vi "~Graph Sequence test.vi"(10 "PAARD Test Seq":T1[](array[typedef])=[{"StepType"=enum."Motion", "RF In/Out"=enum."Rx - RF Out", "Module/Raster"=0, "Polarization"=enum."Horizontal", "AO-64 Array"=[], "Position"=[]}, {"StepType"=enum."RasterTest", "RF In/Out"=enum."Tx - RF In", "Module/Raster"=0, "Polarization"=enum."Vertical", "AO-64 Array"=[], "Position"=[]}, {"StepType"=enum."Motion", "RF In/Out"=enum."Rx - RF Out", "Module/Raster"=1, "Polarization"=enum."Horizontal", "AO-64 Array"=[], "Position"=[]}, {"StepType"=enum."RasterTest", "RF In/Out"=enum."Tx - RF In", "Module/Raster"=0, "Polarization"=enum."Vertical", "AO-64 Array"=[], "Position"=[]}, {"StepType"=enum."Motion", "RF In/Out"=enum."Rx - RF Out", "Module/Raster"=2, "Polarization"=enum."Horizontal", "AO-64 Array"=[], "Position"=[]}, {"StepType"=enum."RasterTest", "RF In/Out"=enum."Tx - RF In", "Module/Raster"=0, "Polarization"=enum."Vertical", "AO-64 Array"=[], "Position"=[]}, {"StepType"=enum."Motion", "RF In/Out"=enum."Rx - RF Out", "Module/Raster"=3, "Polarization"=enum."Horizontal", "AO-64 Array"=[], "Position"=[]}, {"StepType"=enum."RasterTest", "RF In/Out"=enum."Tx - RF In", "Module/Raster"=0, "Polarization"=enum."Vertical", "AO-64 Array"=[], "Position"=[]}, {"StepType"=enum."Motion", "RF In/Out"=enum."Rx - RF Out", "Module/Raster"=4, "Polarization"=enum."Horizontal", "AO-64 Array"=[], "Position"=[]}, {"StepType"=enum."RasterTest", "RF In/Out"=enum."Tx - RF In", "Module/Raster"=0, "Polarization"=enum."Vertical", "AO-64 Array"=[], "Position"=[]}, {"StepType"=enum."Motion", "RF In/Out"=enum."Rx - RF Out", "Module/Raster"=5, "Polarization"=enum."Horizontal", "AO-64 Array"=[], "Position"=[]}, {"StepType"=enum."RasterTest", "RF In/Out"=enum."Tx - RF In", "Module/Raster"=0, "Polarization"=enum."Vertical", "AO-64 Array"=[], "Position"=[]}, {"StepType"=enum."Motion", "RF In/Out"=enum."Rx - RF Out", "Module/Raster"=6, "Polarization"=enum."Horizontal", "AO-64 Array"=[], "Position"=[]}, {"StepType"=enum."RasterTest", "RF In/Out"=enum."Tx - RF In", "Module/Raster"=0, "Polarization"=enum."Vertical", "AO-64 Array"=[], "Position"=[]}, {"StepType"=enum."Motion", "RF In/Out"=enum."Rx - RF Out", "Module/Raster"=7, "Polarization"=enum."Horizontal", "AO-64 Array"=[], "Position"=[]}, {"StepType"=enum."RasterTest", "RF In/Out"=enum."Tx - RF In", "Module/Raster"=0, "Polarization"=enum."Vertical", "AO-64 Array"=[], "Position"=[]}, {"StepType"=enum."Motion", "RF In/Out"=enum."Rx - RF Out", "Module/Raster"=8, "Polarization"=enum."Horizontal", "AO-64 Array"=[], "Position"=[]}, {"StepType"=enum."RasterTest", "RF In/Out"=enum."Tx - RF In", "Module/Raster"=0, "Polarization"=enum."Vertical", "AO-64 Array"=[], "Position"=[]}, {"StepType"=enum."Motion", "RF In/Out"=enum."Rx - RF Out", "Module/Raster"=9, "Polarization"=enum."Horizontal", "AO-64 Array"=[], "Position"=[]}, {"StepType"=enum."RasterTest", "RF In/Out"=enum."Tx - RF In", "Module/Raster"=0, "Polarization"=enum."Vertical", "AO-64 Array"=[], "Position"=[]}, {"StepType"=enum."Motion", "RF In/Out"=enum."Rx - RF Out", "Module/Raster"=10, "Polarization"=enum."Horizontal", "AO-64 Array"=[], "Position"=[]}, {"StepType"=enum."RasterTest", "RF In/Out"=enum."Tx - RF In", "Module/Raster"=0, "Polarization"=enum."Vertical", "AO-64 Array"=[], "Position"=[]}, {"StepType"=enum."Motion", "RF In/Out"=enum."Rx - RF Out", "Module/Raster"=11, "Polarization"=enum."Horizontal", "AO-64 Array"=[], "Position"=[]}, {"StepType"=enum."RasterTest", "RF In/Out"=enum."Tx - RF In", "Module/Raster"=0, "Polarization"=enum."Vertical", "AO-64 Array"=[], "Position"=[]}, {"StepType"=enum."Motion", "RF In/Out"=enum."Rx - RF Out", "Module/Raster"=12, "Polarization"=enum."Horizontal", "AO-64 Array"=[], "Position"=[]}, {"StepType"=enum."RasterTest", "RF In/Out"=enum."Tx - RF In", "Module/Raster"=0, "Polarization"=enum."Vertical", "AO-64 Array"=[], "Position"=[]}, {"StepType"=enum."Motion", "RF In/Out"=enum."Rx - RF Out", "Module/Raster"=13, "Polarization"=enum."Horizontal", "AO-64 Array"=[], "Position"=[]}, {"StepType"=enum."RasterTest", "RF In/Out"=enum."Tx - RF In", "Module/Raster"=0, "Polarization"=enum."Vertical", "AO-64 Array"=[], "Position"=[]}, {"StepType"=enum."Motion", "RF In/Out"=enum."Rx - RF Out", "Module/Raster"=14, "Polarization"=enum."Horizontal", "AO-64 Array"=[], "Position"=[]}, {"StepType"=enum."RasterTest", "RF In/Out"=enum."Tx - RF In", "Module/Raster"=0, "Polarization"=enum."Vertical", "AO-64 Array"=[], "Position"=[]}, {"StepType"=enum."Motion", "RF In/Out"=enum."Rx - RF Out", "Module/Raster"=15, "Polarization"=enum."Horizontal", "AO-64 Array"=[], "Position"=[]}, {"StepType"=enum."RasterTest", "RF In/Out"=enum."Tx - RF In", "Module/Raster"=0, "Polarization"=enum."Vertical", "AO-64 Array"=[], "Position"=[]}, {"StepType"=enum."Motion", "RF In/Out"=enum."Rx - RF Out", "Module/Raster"=16, "Polarization"=enum."Horizontal", "AO-64 Array"=[], "Position"=[]}, {"StepType"=enum."RasterTest", "RF In/Out"=enum."Tx - RF In", "Module/Raster"=0, "Polarization"=enum."Vertical", "AO-64 Array"=[], "Position"=[]}, {"StepType"=enum."Motion", "RF In/Out"=enum."Rx - RF Out", "Module/Raster"=17, "Polarization"=enum."Horizontal", "AO-64 Array"=[], "Position"=[]}, {"StepType"=enum."RasterTest", "RF In/Out"=enum."Tx - RF In", "Module/Raster"=0, "Polarization"=enum."Vertical", "AO-64 Array"=[], "Position"=[]}, {"StepType"=enum."Motion", "RF In/Out"=enum."Rx - RF Out", "Module/Raster"=18, "Polarization"=enum."Horizontal", "AO-64 Array"=[], "Position"=[]}, {"StepType"=enum."RasterTest", "RF In/Out"=enum."Tx - RF In", "Module/Raster"=0, "Polarization"=enum."Vertical", "AO-64 Array"=[], "Position"=[]}, {"StepType"=enum."Motion", "RF In/Out"=enum."Rx - RF Out", "Module/Raster"=19, "Polarization"=enum."Horizontal", "AO-64 Array"=[], "Position"=[]}, {"StepType"=enum."RasterTest", "RF In/Out"=enum."Tx - RF In", "Module/Raster"=0, "Polarization"=enum."Vertical", "AO-64 Array"=[], "Position"=[]}, {"StepType"=enum."Finish", "RF In/Out"=enum."Tx - RF In", "Module/Raster"=0, "Polarization"=enum."Vertical", "AO-64 Array"=[], "Position"=[]}]) -> ()   [LabVIEW 2018]
uses:
  mWaveTestStep.ctl
  TestStepTypes.ctl
  RF Direction.ctl
  PolarizationSelect.ctl
  APARMainSubvis/VXM Public API/singleAxisMoveDef.ctl
  APARMainSubvis/VXM Public API/mmWaveAxis.ctl
panel:
  out "Waveform Graph":i32[][](graph)
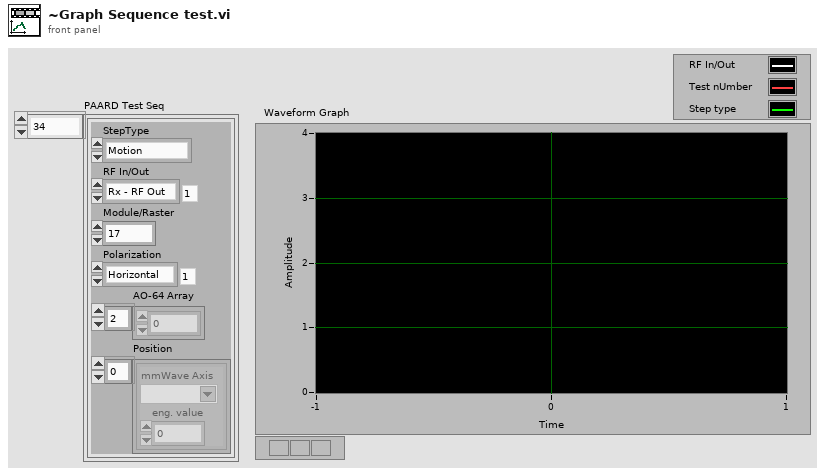
[diagram p1: front panel]
types:
  T1 = typedef "mWaveTestStep.ctl" = cluster{"StepType":T2, "RF In/Out":T3, "Module/Raster":i32, "Polarization":T4, "AO-64 Array":dbl[], "Position":T5[]}
  T2 = typedef "TestStepTypes.ctl" = enum16{"MotionFF-M2", "Motion", "SweepTest", "RasterTest", "Finish", "64ModuleCfg"}
  T3 = typedef "RF Direction.ctl" = enum16{"Tx - RF In", "Rx - RF Out"}
  T4 = typedef "PolarizationSelect.ctl" = enum16{"Vertical", "Horizontal"}
  T5 = typedef "singleAxisMoveDef.ctl" = cluster{"mmWave Axis":T6, "eng. value":dbl}
  T6 = typedef "mmWaveAxis.ctl" = string
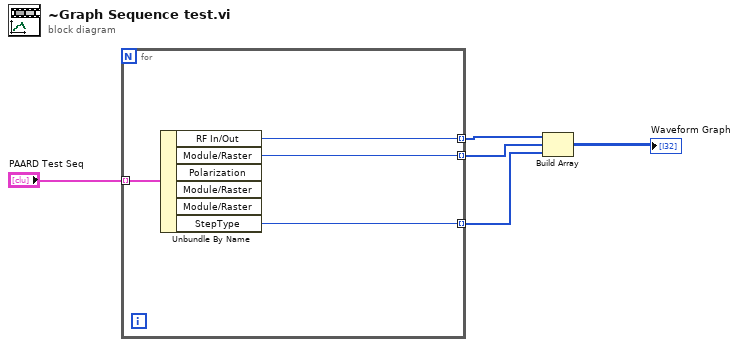
[diagram p0: block diagram]
diagram:
  n1 = for {
    tunnel: "PAARD Test Seq" -> [w9] mode=indexing
    tunnel: [w8] -> w4 mode=indexing
    tunnel: [w7] -> w3 mode=indexing
    tunnel: [w6] -> w2 mode=indexing
    n2 = Unbundle By Name(w9) -> ("RF In/Out"=w8:T3, "Module/Raster"=w7:i32, "StepType"=w6:T2)  [unwired: 3 out]
  }
  n3 = Build Array(w4, w3, w2) -> (→"Waveform Graph":i32[][])
